vi "PostRoom.vi"(7 "LabVIEW Web Service Request":refnum<class "Web Request.lvclass">, 8 "Data":string, 9 "Command":string, 10 "Room":i32) -> (1 "Response":string)   [LabVIEW 2015]
uses:
  <vilib>/wsapi/Web Request.lvclass
  TypeDef/RoomsActionEnum.ctl
  TypeDef/RequestActionEnum.ctl
  LVClasses/Request/Request.lvclass/Request.ctl
  LVClasses/Request/Read Summary.vi
  LVClasses/Request/Request.lvclass
panel:
  out "current time":timestamp
  out "request variables":cluster{"Key":string[], "Value":string[]}
  out "postdata":string
  # "Use the Web Service Request input terminal to call the VIs on the Web Services palette. Do not remove it from the connector pane unless you don't need access to the palette."
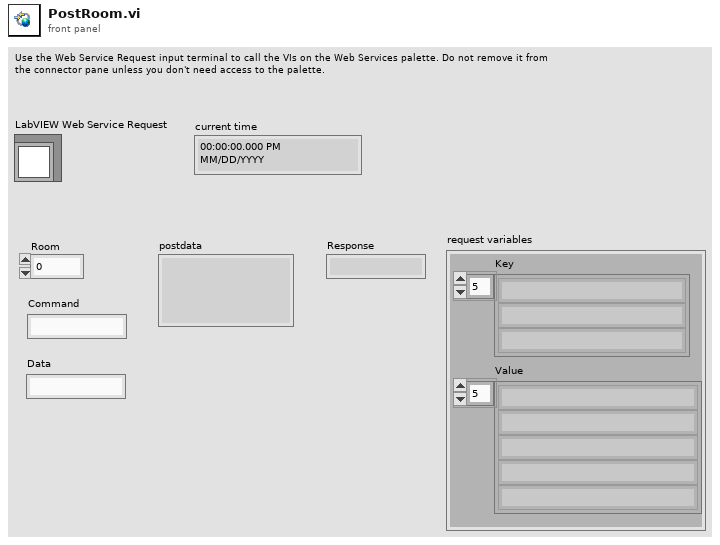
[diagram p1: front panel]
types:
  T1 = typedef "RoomsActionEnum.ctl" = enum16{"Init", "Add Room", "Remove Room", "Read Room", "Read Flag", "Read Flag State", "Write Flag State", "Read Flag Color", "Write Flag Color", "Read Bed Vacant", "Write Bed Vacant", "Read Personnel", "Add Personnel", "Remove Personnel", "Read Requests", "Add Request", "Remove Request", "Read Beacon ID", "Write Beacon ID", "Write Bed URL", "Read Bed URL", "Read Rooms Numbers", "Write Flag"}
  T2 = typedef "RequestActionEnum.ctl" = enum16{"Init", "ReadRequests", "ReadRequest", "AddRequest", "RemoveRequest", "ToDisk", "Ack", "Complete", "CheckAlarms", "PIntoRoom", "Read Summary"}
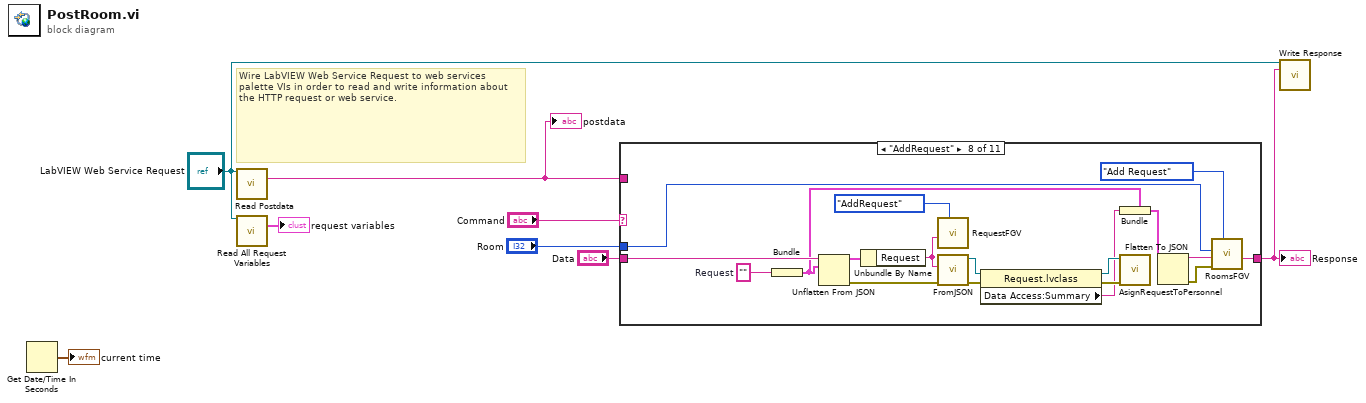
[diagram p0: block diagram]
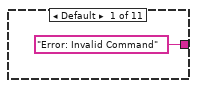
[diagram p2: hidden frame]
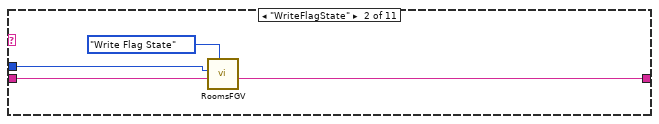
[diagram p3: hidden frame]
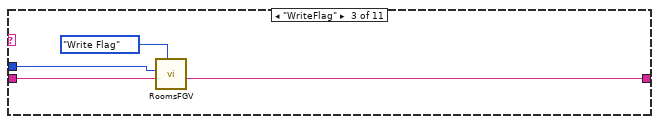
[diagram p4: hidden frame]
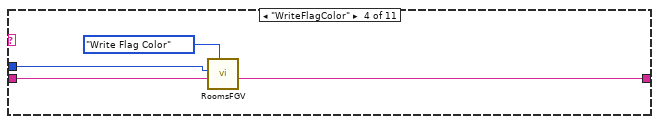
[diagram p5: hidden frame]
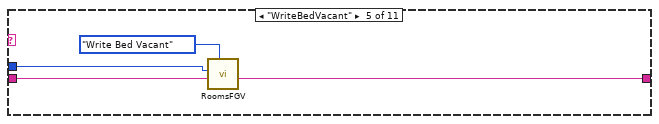
[diagram p6: hidden frame]
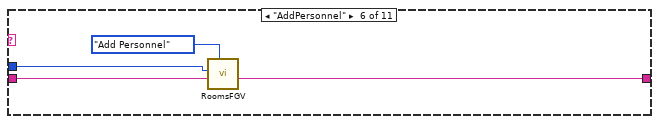
[diagram p7: hidden frame]
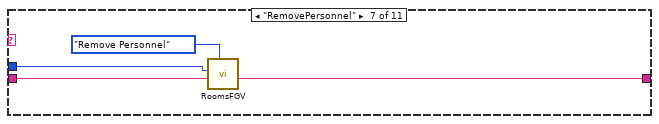
[diagram p8: hidden frame]
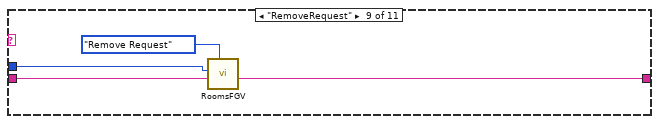
[diagram p9: hidden frame]
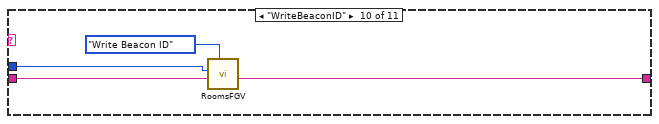
[diagram p10: hidden frame]
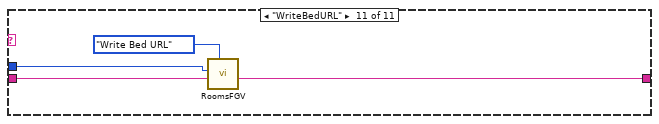
[diagram p11: hidden frame]
diagram:
  # "Wire LabVIEW Web Service Request to web services palette VIs in order to read and write information about the HTTP request or web service."
  n1 = Get Date/Time In Seconds() -> (seconds since 1Jan1904=→"current time":timestamp)
  n2 = call <vilib>:"Read Postdata.vi"("LabVIEW Web Service Request"="LabVIEW Web Service Request") -> ("postdata"=w7:string)  [unwired: 12 in, 2 out]
  "postdata" <- w7
  n3 = call <vilib>:"Read All Request Variables.vi"("LabVIEW Web Service Request"="LabVIEW Web Service Request") -> ("request variables"=→"request variables":cluster{"Key":string[], "Value":string[]})  [unwired: 12 in, 2 out]
  n4 = case shown="\"AddRequest\"" "Command" {
    tunnel: w7 -> [_ _ _ _ _ _ _ _ _ _ _]
    tunnel: ["Error: Invalid Command" ("Data Out") w12 w17 w20 w24 w28 w32 w50 w54 w58 w62] -> w3
    tunnel: "Room" -> [_ w11 w16 w19 w23 w27 w31 w49 w53 w57 w61]
    tunnel: "Data" -> [_ w10 w15 w18 w22 w26 w30 w43 w52 w56 w60]
    frame Default {
    }
    frame "WriteFlagState" {
      n5 = call "RoomsFGV.vi"("Actions"=RoomsActionEnum."Write Flag State", "Data In"=w10, "Room"=w11) -> ("Data Out"=w12:string)  [unwired: 7 in, 1 out]
    }
    frame "WriteFlag" {
      n6 = call "RoomsFGV.vi"("Actions"=RoomsActionEnum."Write Flag", "Data In"=w15, "Room"=w16) -> ("Data Out"=w17:string)  [unwired: 7 in, 1 out]
    }
    frame "WriteFlagColor" {
      n7 = call "RoomsFGV.vi"("Actions"=RoomsActionEnum."Write Flag Color", "Data In"=w18, "Room"=w19) -> ("Data Out"=w20:string)  [unwired: 7 in, 1 out]
    }
    frame "WriteBedVacant" {
      n8 = call "RoomsFGV.vi"("Actions"=RoomsActionEnum."Write Bed Vacant", "Data In"=w22, "Room"=w23) -> ("Data Out"=w24:string)  [unwired: 7 in, 1 out]
    }
    frame "AddPersonnel" {
      n9 = call "RoomsFGV.vi"("Actions"=RoomsActionEnum."Add Personnel", "Data In"=w26, "Room"=w27) -> ("Data Out"=w28:string)  [unwired: 7 in, 1 out]
    }
    frame "RemovePersonnel" {
      n10 = call "RoomsFGV.vi"("Actions"=RoomsActionEnum."Remove Personnel", "Data In"=w30, "Room"=w31) -> ("Data Out"=w32:string)  [unwired: 7 in, 1 out]
    }
    frame "AddRequest" {
      w46 = ""  # Request
      n11 = Bundle("Request"=w46) -> (w41:cluster{"Request":string})  [unwired: 1 in]
      n12 = Unflatten From JSON(JSON string=w43, type and defaults=w41) -> (value=w45:cluster{"Request":string}, error out=w47:errorcluster)  [unwired: 5 in]
      n13 = Unbundle By Name(w45) -> ("Request"=w44:string)
      n14 = call "RequestFGV.vi"("Actions"=RequestActionEnum."AddRequest", "Data In"=w44) -> ()  [unwired: 8 in, 2 out]
      n15 = call "FromJSON.vi"("error in (no error)"=w47, "Request"=w44) -> ("error out"=w39:errorcluster, "Request out"=w40:refnum<class "Request.lvclass">)  [unwired: 8 in]
      n16 = property class="Request.lvclass"(reference=w40, error in=w39) -> (reference out=w37:refnum<class "Request.lvclass">, error out=w38:errorcluster, "Data Access:Summary"=w36:string)
      n17 = Bundle(cluster=w41, "Request"=w36) -> (w42:cluster{"Request":string})
      n18 = call "AsignRequestToPersonnel.vi"("error in (no error)"=w38, "Request in"=w37) -> ()  [unwired: 9 in, 1 out]
      n19 = Flatten To JSON(anything=w42) -> (JSON string=w35:string, 11:w34:errorcluster)  [unwired: 2 in]
      n20 = call "RoomsFGV.vi"("Actions"=RoomsActionEnum."Add Request", "error in (no error)"=w34, "Data In"=w35, "Room"=w49) -> ("Data Out"=w50:string)  [unwired: 6 in, 1 out]
    }
    frame "RemoveRequest" {
      n21 = call "RoomsFGV.vi"("Actions"=RoomsActionEnum."Remove Request", "Data In"=w52, "Room"=w53) -> ("Data Out"=w54:string)  [unwired: 7 in, 1 out]
    }
    frame "WriteBeaconID" {
      n22 = call "RoomsFGV.vi"("Actions"=RoomsActionEnum."Write Beacon ID", "Data In"=w56, "Room"=w57) -> ("Data Out"=w58:string)  [unwired: 7 in, 1 out]
    }
    frame "WriteBedURL" {
      n23 = call "RoomsFGV.vi"("Actions"=RoomsActionEnum."Write Bed URL", "Data In"=w60, "Room"=w61) -> ("Data Out"=w62:string)  [unwired: 7 in, 1 out]
    }
  }
  "Response" <- w3
  n24 = call <vilib>:"Write Response.vi"("LabVIEW Web Service Request"="LabVIEW Web Service Request", "response string"=w3) -> ()  [unwired: 12 in, 2 out]
